vi "Unit Tests.vi"   [LabVIEW 2019]
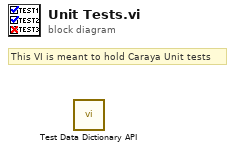
[diagram p0: block diagram]
diagram:
  # "This VI is meant to hold Caraya Unit tests"
  n1 = call "Test Data Dictionary API.vi"() -> ()  [unwired: 11 in, 1 out]
